vi "CSV1_setup (SubVI).vi"(8 "error in (no error)":errorcluster, 9 "append to file? (new file:F)":bool, 10 "prompt":string, 11 "file path (dialog if empty)":path) -> (0 "error out":errorcluster, 3 "file refnum out":refnum<file>)   [LabVIEW 2012]
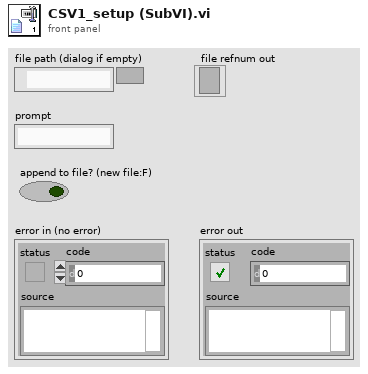
[diagram p1: front panel]
types:
  T1 = enum16{"open", "replace", "create", "open or create", "replace or create", "replace or create with confirmation"}
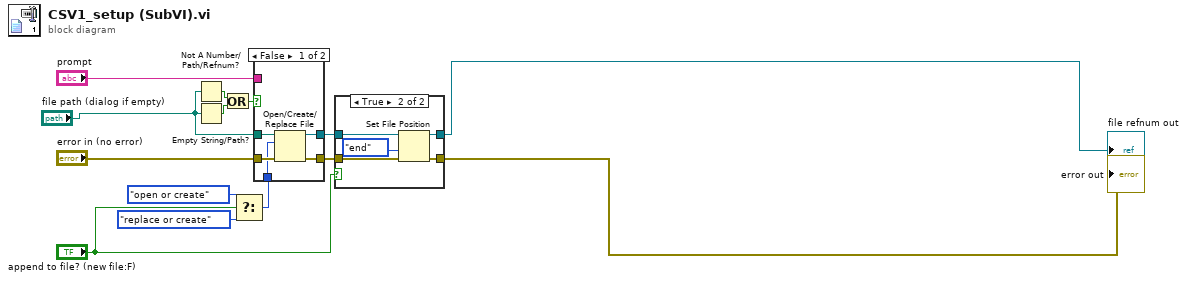
[diagram p0: block diagram]
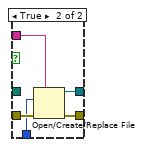
[diagram p3: hidden frame]
diagram:
  n1 = Not A Number/Path/Refnum?(number/path/refnum="file path (dialog if empty)") -> (NaN/Path/Refnum?=w4:bool)
  n2 = Empty String/Path?(string/path="file path (dialog if empty)") -> (empty?=w3:bool)
  n3 = Or(x=w4, y=w3) -> (x .or. y?=w5:bool)
  n4 = Select ("function")(t=T1."open or create" ("operation (0:open)"), s="append to file? (new file:F)", f=T1."replace or create" ("operation (0:open)")) -> (s? t:f=w8:T1)
  n5 = case shown="False" w5 {
    tunnel: "prompt" -> [_ w22]
    tunnel: "error in (no error)" -> [w19 w23]
    tunnel: [w18 w24] -> w9
    tunnel: [w17 w21] -> w10
    tunnel: "file path (dialog if empty)" -> [w16 _]
    tunnel: w8 -> [w15 w20]
    frame False {
      n6 = Open/Create/Replace File(file path (use dialog)=w16, error in=w19, operation (0:open)=w15) -> (refnum out=w17:refnum<file>, error out=w18:errorcluster)  [unwired: 3 in, 1 out]
    }
    frame True {
      n7 = Open/Create/Replace File(error in=w23, prompt=w22, operation (0:open)=w20) -> (refnum out=w21:refnum<file>, error out=w24:errorcluster)  [unwired: 3 in, 1 out]
    }
  }
  n8 = case shown="True" "append to file? (new file:F)" {
    tunnel: w9 -> [w25 w31]
    tunnel: [w25 w30] -> w13
    tunnel: w10 -> [w26 w28]
    tunnel: [w26 w29] -> w12
    frame False {
    }
    frame True {
      n9 = Set File Position(refnum=w28, from (0:start)=enum16{"start", "end", "current"}."end", error in=w31) -> (refnum out=w29:refnum<file>, error out=w30:errorcluster)  [unwired: 1 in]
    }
  }
  "error out" <- w13
  "file refnum out" <- w12
